vi "Close_core.vi"(8 "error in (no error)":errorcluster, 11 "CtlReferences in":refnum<class "CtlReferences.lvclass">) -> (0 "error out":errorcluster)   [LabVIEW 2020, in "CtlReferences.lvlib" / "CtlReferences.lvclass"]
uses:
  CtlReferences.lvclass
  CtlReferences.lvclass/CtlReferences.ctl
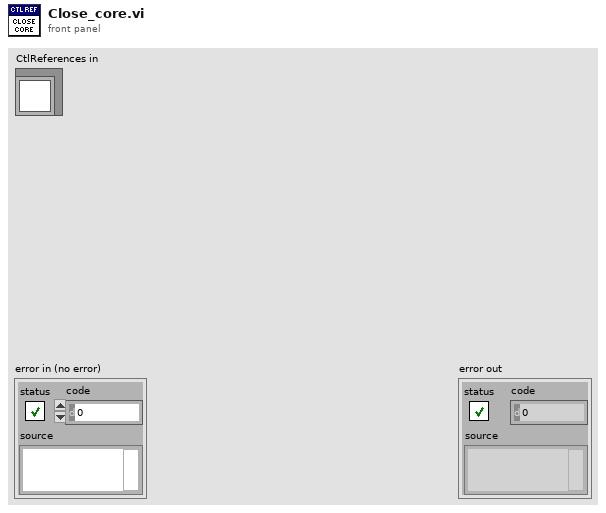
[diagram p1: front panel]
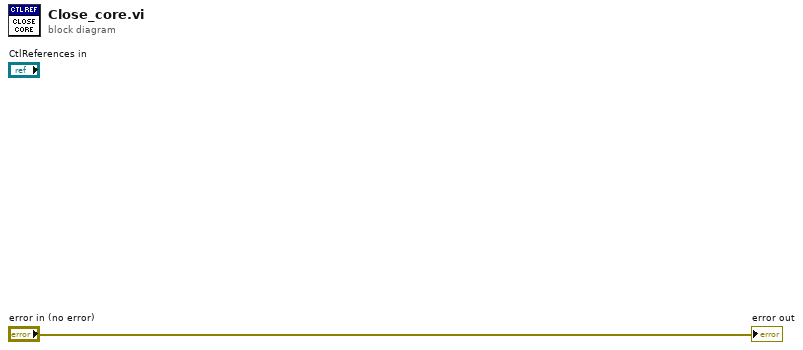
[diagram p0: block diagram]
diagram:
  "error out" <- "error in (no error)"
